vi "LEDTest.vi"() -> ()   [LabVIEW 2019]
panel:
  in  "Color 2":enum16{"Green", "Red", "Dimm"}(ring)=enum."Dimm"
  in  "Color":enum16{"Green", "Red", "Dimm"}(ring)
  in  "Stop Button":bool
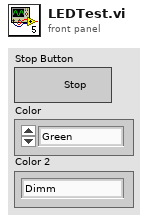
[diagram p1: front panel]
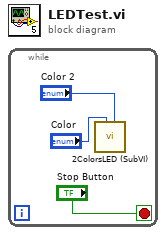
[diagram p0: block diagram]
diagram:
  n1 = while {
    stop <- "Stop Button" stop-if-true
    n2 = call "2ColorsLED (SubVI).vi"("Color 2"="Color 2", "Color"="Color") -> ()  [unwired: 9 in, 1 out]
  }
